vi "elektrische-Leistung.vi"(10 "Dynamic Data":dynamicdata(waveform), 11 "Dynamic Data 2":dynamicdata(waveform)) -> (3 "Elektrische Leistung":waveform(dbl)(graph))   [LabVIEW 2018]
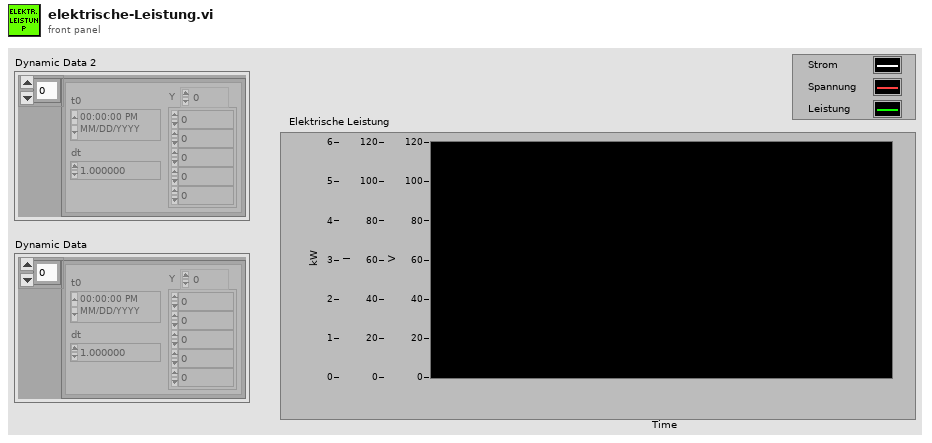
[diagram p1: front panel]
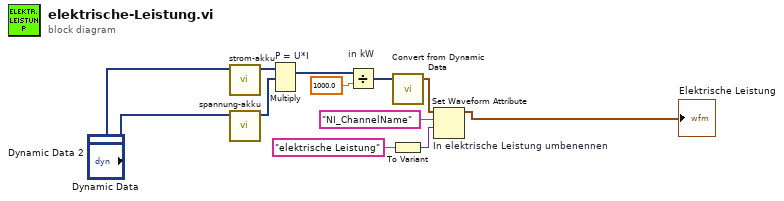
[diagram p0: block diagram]
diagram:
  n1 = call "strom-akku.vi"("Dynamic Data"="Dynamic Data 2") -> ("Filtered Signal"=w4:dynamicdata)  [unwired: 10 in]
  n2 = call "spannung-akku.vi"("Dynamic Data in"="Dynamic Data") -> ("Dynamic Data out"=w3:dynamicdata)  [unwired: 10 in]
  n3 = Multiply "P = U*I"(1:w3, 2:w4) -> (0:w6:dynamicdata)  [unwired: 1 in, 1 out]
  n4 = Divide "in kW"(x=w6, y=1000.0) -> (x/y=w7:dynamicdata)
  n5 = call "Convert from Dynamic Data"("Dynamic Data Type"=w7) -> ("Waveform"=w8:waveform(dbl))  [unwired: 3 in]
  n6 = To Variant(anything="elektrische Leistung") -> (Variant=w11:variant)
  n7 = Set Waveform Attribute "In elektrische Leistung umbenennen"(5:w11, 6:"NI_ChannelName" ("name"), 7:w8) -> (3:→"Elektrische Leistung":waveform(dbl))  [unwired: 1 in, 2 out]
